vi "Preview Control States.vi"(8 "error in":errorcluster, 11 "Control in":refnum<class "Control.lvclass">) -> (0 "error out":errorcluster, 2 "States preview":picture[](array[picture]), 3 "Control out":refnum<class "Control.lvclass">)   [LabVIEW 2012, in "Control.lvclass"]
uses:
  Control.lvclass
  Control.lvclass/Control.ctl
  <userlib>/BitMan/BitMap class/BitMap.lvclass
  <userlib>/BitMan/Built-in Filters class/Built-in Filters.lvclass
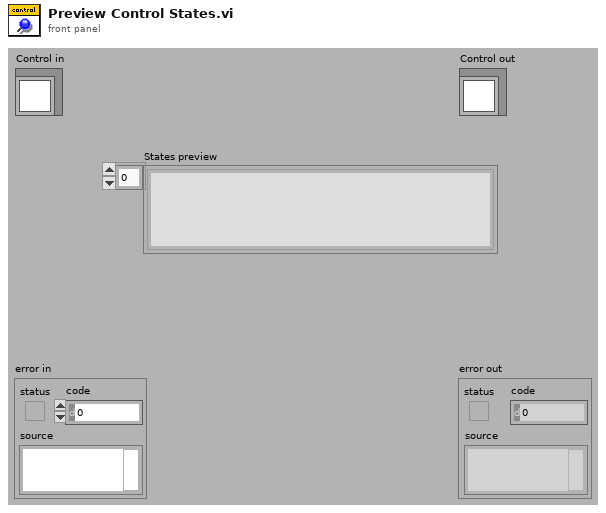
[diagram p1: front panel]
types:
  T1 = enum16{"User-specified Font", "Application Font", "System Font", "Dialog Font"}
  T2 = typedef "Control.lvclass/BX.Orientation__LCR _Modified.ctl" = u8
  T3 = typedef "Control.lvclass/_ui_tools_font.ctl" = cluster{"Font Name:":string, "Size":i16, "Strikeout?":bool, "Italic?":bool, "Underline?":bool, "Outline?":bool, "Shadow?":bool, "Bold?":bool}
  T4 = typedef "imagedata.ctl" = cluster{"image type":i32, "image depth":i32, "image":u8[], "mask":u8[], "colors":u32[], "Rectangle":cluster{"left":i16, "top":i16, "right":i16, "bottom":i16}}
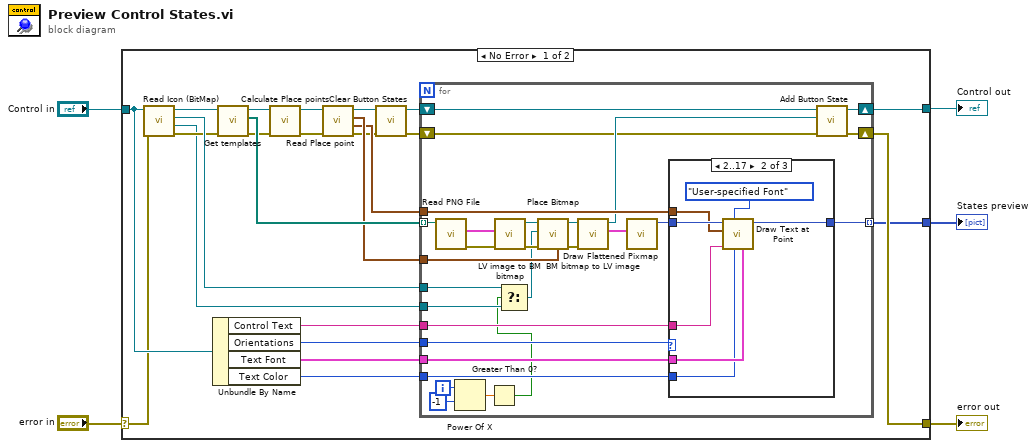
[diagram p0: block diagram]
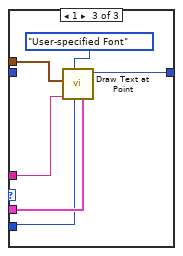
[diagram p3: hidden frame]
diagram:
  n1 = case shown="No Error" "error in" {
    selector: "error in" -> [w14 w73]
    tunnel: [w21 w73] -> w4
    tunnel: [w22 w72] -> w2
    tunnel: "Control in" -> [w18 w72]
    tunnel: [w20 _] -> w1
    frame No Error {
      n2 = call-dynamic "Read Icon (BitMap).vi"("error in (no error)"=w14, "Control in"=w18) -> ("error out"=w15:errorcluster, "Icon (BitMap) True"=w6:refnum<class "BitMap.lvclass">, "Icon (BitMap) False"=w26:refnum<class "BitMap.lvclass">, "Control out"=w16:refnum<class "Control.lvclass">)  [unwired: 6 out]
      n3 = Unbundle By Name(w18) -> ("Control Text"=w17:string, "Orientations"=w19:T2, "Text Font"=w9:T3, "Text Color"=w7:u32)
      n4 = call-dynamic "Get templates.vi"("error in (no error)"=w15, "Control in"=w16) -> ("error out"=w13:errorcluster, "PNG templates"=w29:path[], "Control out"=w8:refnum<class "Control.lvclass">)  [unwired: 7 out]
      n5 = call-dynamic "Calculate Place points.vi"("error in (no error)"=w13, "Control in"=w8) -> ("error out"=w12:errorcluster, "Control out"=w27:refnum<class "Control.lvclass">)  [unwired: 8 out]
      n6 = call-dynamic "Read Place point.vi"("error in (no error)"=w12, "Control in"=w27) -> ("error out"=w10:errorcluster, "Text Point"=w25:cluster{"x":i32, "y":i32}, "Point"=w28:cluster{"x":i32, "y":i32}, "Control out"=w11:refnum<class "Control.lvclass">)  [unwired: 6 out]
      n7 = call-dynamic "Clear Button States.vi"("error in (no error)"=w10, "Control in"=w11) -> ("error out"=w23:errorcluster, "Control out"=w24:refnum<class "Control.lvclass">)  [unwired: 8 out]
      n8 = for {
        tunnel: w29 -> [w52] mode=indexing
        tunnel: [w46] -> w20 mode=indexing
        tunnel: w28 -> [w51]
        tunnel: w26 -> [w35]
        tunnel: w17 -> [w48]
        tunnel: w25 -> [w45]
        shift-right: [w43] -> w22
        shift-left: w24 -> [w44]
        shift-right: [w41] -> w21
        shift-left: w23 -> [w40]
        tunnel: w19 -> [w39]
        tunnel: w9 -> [w38]
        tunnel: w7 -> [w37]
        tunnel: w6 -> [w36]
        i -> [w33]
        n9 = call <vilib>:"Read PNG File.vi"("path to PNG file"=w52) -> ("error out"=w57:errorcluster, "image data"=w56:T4)  [unwired: 1 in, 8 out]
        n10 = Power Of X(1:-1 ("x"), 2:w33) -> (0:w31:dbl)
        n11 = Greater Than 0?(x=w31) -> (x > 0?=w30:bool)
        n12 = call <userlib>:"LV image to BM bitmap.vi"("error in (no error)"=w57, "LV image data"=w56) -> ("error out"=w49:errorcluster, "BitMap out"=w50:refnum<class "BitMap.lvclass">)  [unwired: 2 in, 6 out]
        n13 = Select(t=w35, s=w30, f=w36) -> (s? t:f=w34:refnum<class "BitMap.lvclass">)
        n14 = call <userlib>:"Place Bitmap.vi"("Place point"=w51, "error in (no error)"=w49, "Bitmap to place"=w34, "Bitmap in (optional)"=w50) -> ("error out"=w53:errorcluster, "Bitmap out"=w55:refnum<class "BitMap.lvclass">)  [unwired: 2 in, 4 out]
        n15 = call <userlib>:"BM bitmap to LV image.vi"("error in (no error)"=w53, "BitMap in"=w55) -> ("LV image data"=w54:T4, "BitMap out"=w42:refnum<class "BitMap.lvclass">)  [unwired: 1 in, 7 out]
        n16 = call <vilib>:"Draw Flattened Pixmap.vi"("image data"=w54) -> ("new picture"=w47:picture)  [unwired: 1 in, 7 out]
        n17 = case shown="2..17" w39 {
          tunnel: w48 -> [_ w65 w71]
          tunnel: w47 -> [w58 w64 _]
          tunnel: [w58 w63 w70] -> w46
          tunnel: w45 -> [_ w61 w68]
          tunnel: w38 -> [_ w60 w67]
          tunnel: w37 -> [_ w59 w66]
          frame Default {
          }
          frame 2..17 {
            n18 = call <vilib>:"Draw Text at Point.vi"("[user-specified font]"=w60, "text color(black)"=w59, "desired font(Application)"=T1."User-specified Font", "text"=w65, "origin"=w61, "picture"=w64) -> ("new picture"=w63:picture)  [unwired: 3 in, 2 out]
          }
          frame 1 {
            n19 = call <vilib>:"Draw Text at Point.vi"("[user-specified font]"=w67, "text color(black)"=w66, "desired font(Application)"=T1."User-specified Font", "text"=w71, "origin"=w68) -> ("new picture"=w70:picture)  [unwired: 4 in, 2 out]
          }
        }
        n20 = call-dynamic "Add Button State.vi"("error in (no error)"=w40, "State"=w42, "Control in"=w44) -> ("error out"=w41:errorcluster, "Control out"=w43:refnum<class "Control.lvclass">)  [unwired: 7 out]
      }
    }
    frame Error {
    }
  }
  "error out" <- w4
  "Control out" <- w2
  "States preview" <- w1
